vi "Verify CLI Output.vi"(5 "Label":string, 7 "Options":refnum<class "Options.lvclass">, 8 "error in":errorcluster, 9 "CLI Options":T1={"standard input"="", "working directory"=path "", "expected output size  (4096)"=4096, "Run Minimized (T)"=TRUE}, 10 "command line":string, 11 "LUnit Test Case In":refnum<class "Test Case.lvclass">) -> (0 "error out":errorcluster, 3 "LUnit Test Case Out":refnum<class "Test Case.lvclass">)   [LabVIEW 2020, in "LUnit.Extension.lvlib"]
doc: "Uses System Exec to execute command.\n\nCaptures:\nSTD out\nERR out\nReturn Code"
uses:
  LUnit.Extension.lvlib
  <vilib>/Astemes/LUnit/Test Case.lvclass
  Approval Tests/Options/Options.lvclass
  Approval Tests/Verify CLI Options.ctl
  Approval Tests/Options/Options.lvclass/Options.ctl
  Approval Tests/Naming Data/Naming Data.lvclass/Naming Data.ctl
  <vilib>/Astemes/LUnit/Test Case.lvclass/Test Case.ctl
  Approval Tests/Naming Data/Read Test VI Name.vi
  Approval Tests/Naming Data/Write Test VI Name.vi
  <vilib>/Astemes/LUnit/Core/LUnit Test Case/Private/Append Fail Result.vi
  <vilib>/Astemes/LUnit/Core/LUnit Test Case/Private/Append Pass Result.vi
  <vilib>/Astemes/LUnit/Core/LUnit Test Case/Private/Run In UI.vi
  <vilib>/Utility/error.llb/Clear Errors.vi
  Approval Tests/Approval Tests.lvlib
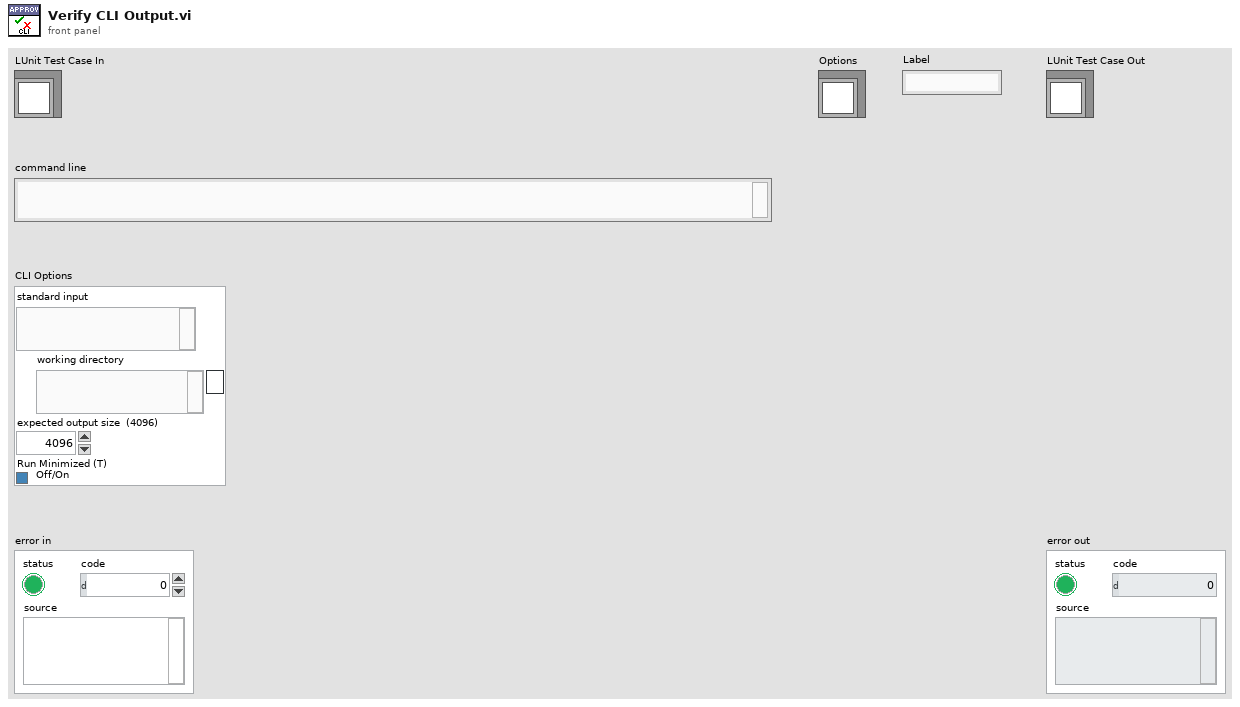
[diagram p1: front panel]
types:
  T1 = typedef "Approval Tests.lvlib/Verify CLI Options.ctl" = cluster{"standard input":string, "working directory":path, "expected output size  (4096)":u32, "Run Minimized (T)":bool}
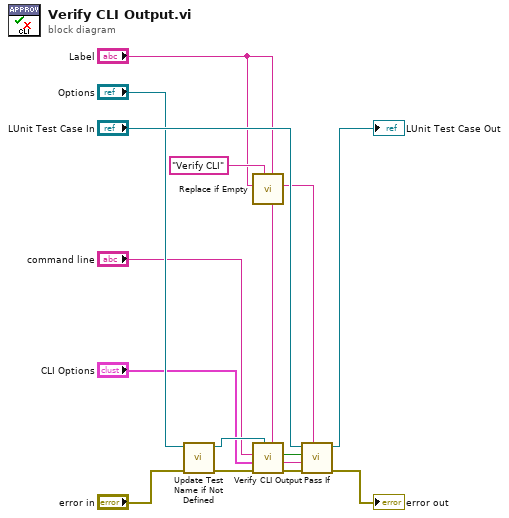
[diagram p0: block diagram]
diagram:
  n1 = call "Update Test Name if Not Defined.vi"("error in"="error in", "Options in"="Options") -> ("error out"=w12:errorcluster, "Options out"=w7:refnum<class "Options.lvclass">)  [unwired: 8 in]
  n2 = call "Replace if Empty.vi"("if empty"="Verify CLI", "Text in"="Label") -> ("Text out"=w1:string)  [unwired: 9 in]
  n3 = call "Verify CLI Output.vi"("Label"="Label", "Approval Tests.lvlib:Options.lvclass"=w7, "error in"=w12, "CLI Options"="CLI Options", "command line"="command line") -> ("error out"=w13:errorcluster, "Failure Message"=w6:string, "Passed?"=w9:bool)  [unwired: 4 in]
  n4 = call <vilib>:"Pass If.vi"("Description"=w1, "error in (no error)"=w13, "Message"=w6, "Pass?"=w9, "LUnit Test Case In"="LUnit Test Case In") -> ("error out"=→"error out":errorcluster, "LUnit Test Case Out"=→"LUnit Test Case Out":refnum<class "Test Case.lvclass">)  [unwired: 5 in]
